vi "Start DAQ.vi"(8 "error in (no error)":errorcluster, 11 "DAQ Interface in":refnum<class "DAQ Interface.lvclass">) -> (0 "error out":errorcluster, 3 "DAQ Interface out":refnum<class "DAQ Interface.lvclass">)   [LabVIEW 2025, in "DAQ Interface.lvlib" / "DAQ Interface.lvclass"]
uses:
  DAQ Interface.lvclass
  DAQ Interface.lvclass/DAQ Interface.ctl
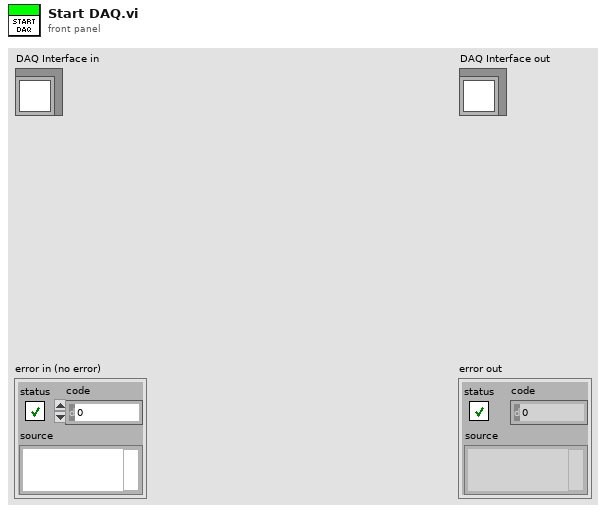
[diagram p1: front panel]
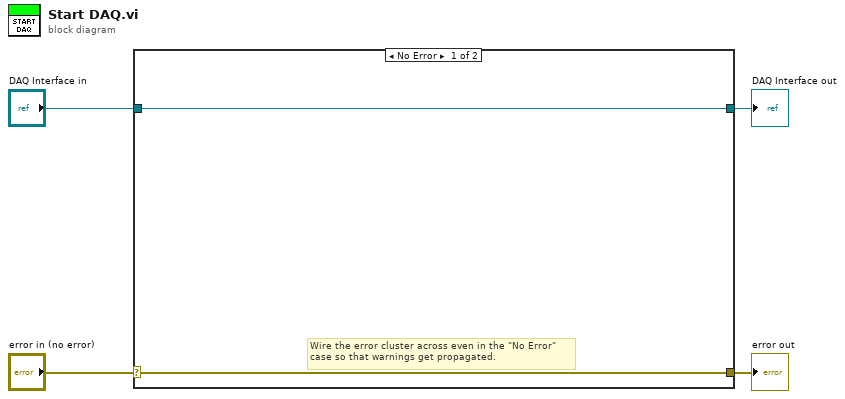
[diagram p0: block diagram]
diagram:
  n1 = case shown="No Error" "error in (no error)" {
    selector: "error in (no error)" -> [w5 w8]
    tunnel: [w5 w8] -> w3
    tunnel: [w6 w7] -> w1
    tunnel: "DAQ Interface in" -> [w6 w7]
    frame No Error {
      # "Wire the error cluster across even in the \"No Error\"\ncase so that warnings get propagated."
    }
    frame Error {
    }
  }
  "error out" <- w3
  "DAQ Interface out" <- w1
